vi "ExeCmd_CallCollect.vi"(4 "HighPrio":bool, 6 "CmdVIRef":refnum<vi>, 7 "ActorClassObjectIn":refnum<class>, 8 "ErrorIn":errorcluster, 9 "NameOfVi2Call(optional)":string, 10 "CmdData":variant, 11 "YActorIn":refnum<class "YActor.lvclass">) -> (0 "ErrorOut":errorcluster, 2 "ReplyData":variant, 5 "ActorClassObjectOut":refnum<class>)   [LabVIEW 2021, in "YActor.lvclass"]
uses:
  YActor.lvclass
  YActor.lvclass/YActor.ctl
  private/CmdCtrl.ctl
  AsyncErrorHandling.ctl
  private/CallMode.ctl
  InlineReferencePool.ctl
panel:
  # "Do not use this VI in a loop where different Cmd VI references are routed.\nThis will cause the execution of the first called command VI only"
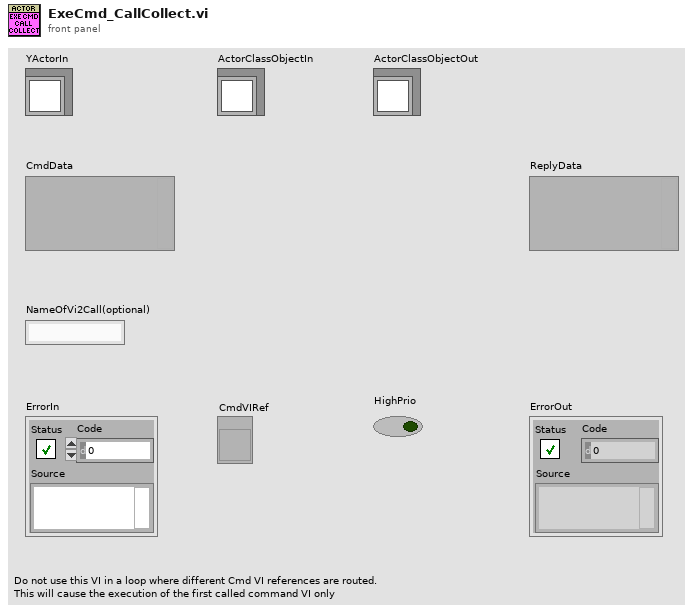
[diagram p1: front panel]
types:
  T1 = typedef "YActor.lvclass/CallMode.ctl" = enum16{"Standard", "Call&Collect"}
  T2 = typedef "YActor.lvclass/InlineReferencePool.ctl" = enum16{"Add", "ClearAll?"}
  T3 = typedef "YActor.lvclass/CmdCtrl.ctl" = cluster{"CmdData":variant, "CommandVI":string, "ReplyQ":i64, "Error":errorcluster, "Msg#":u32, "AsyncErrorHandling":T4, "CallMode":T1, "Source":string}
  T4 = typedef "YActor.lvclass/AsyncErrorHandling.ctl" = enum16{"Return after executing sync command", "Return before executing sync command", "Don't return error"}
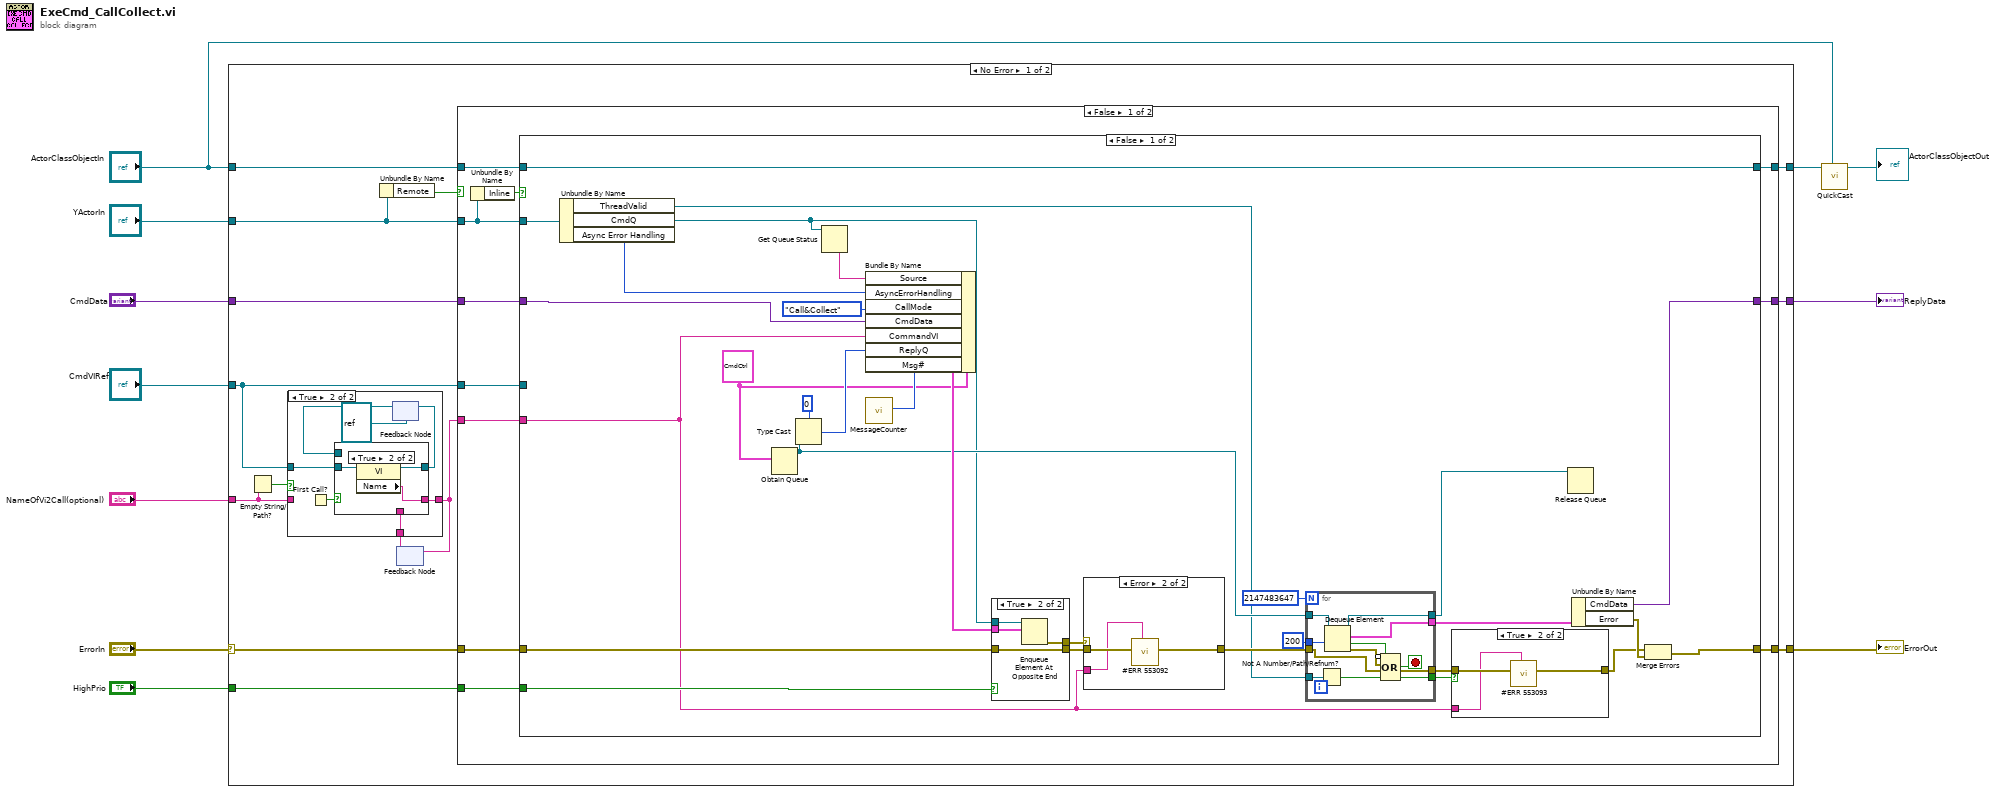
[diagram p0: block diagram]
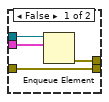
[diagram p6: hidden frame]
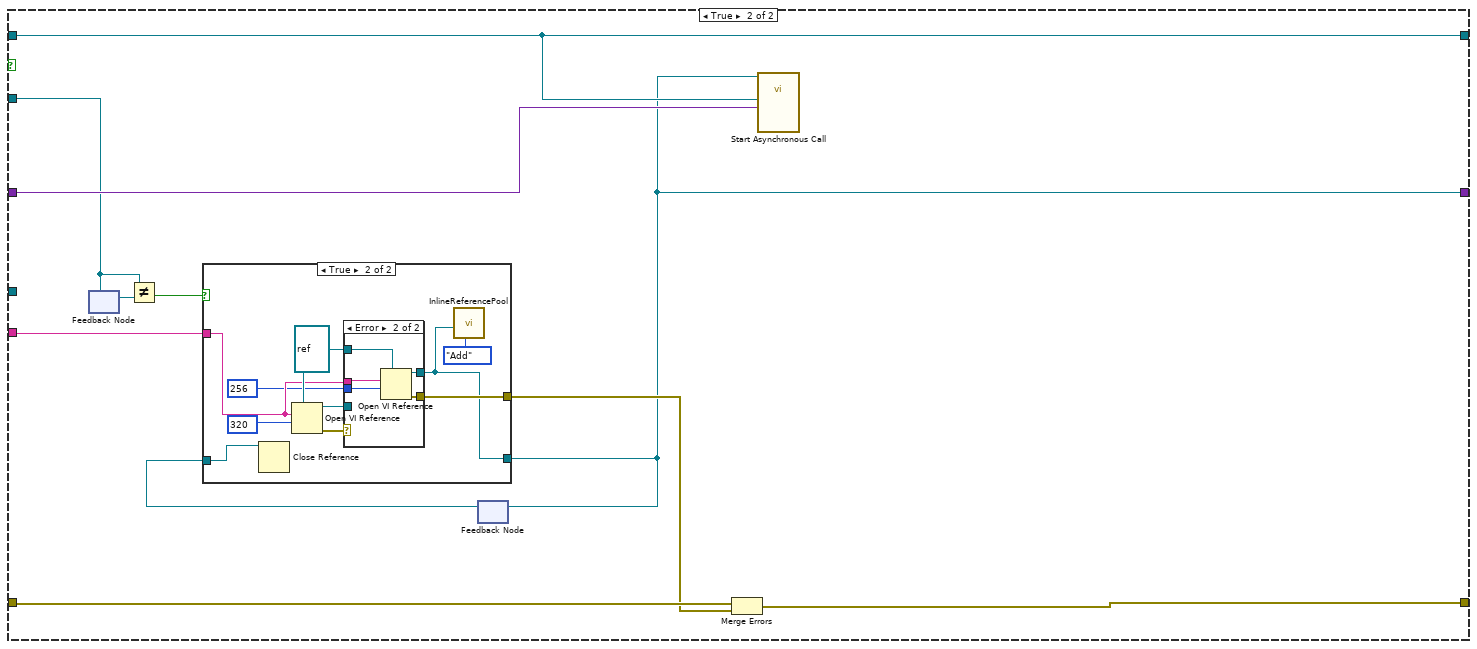
[diagram p7: hidden frame]
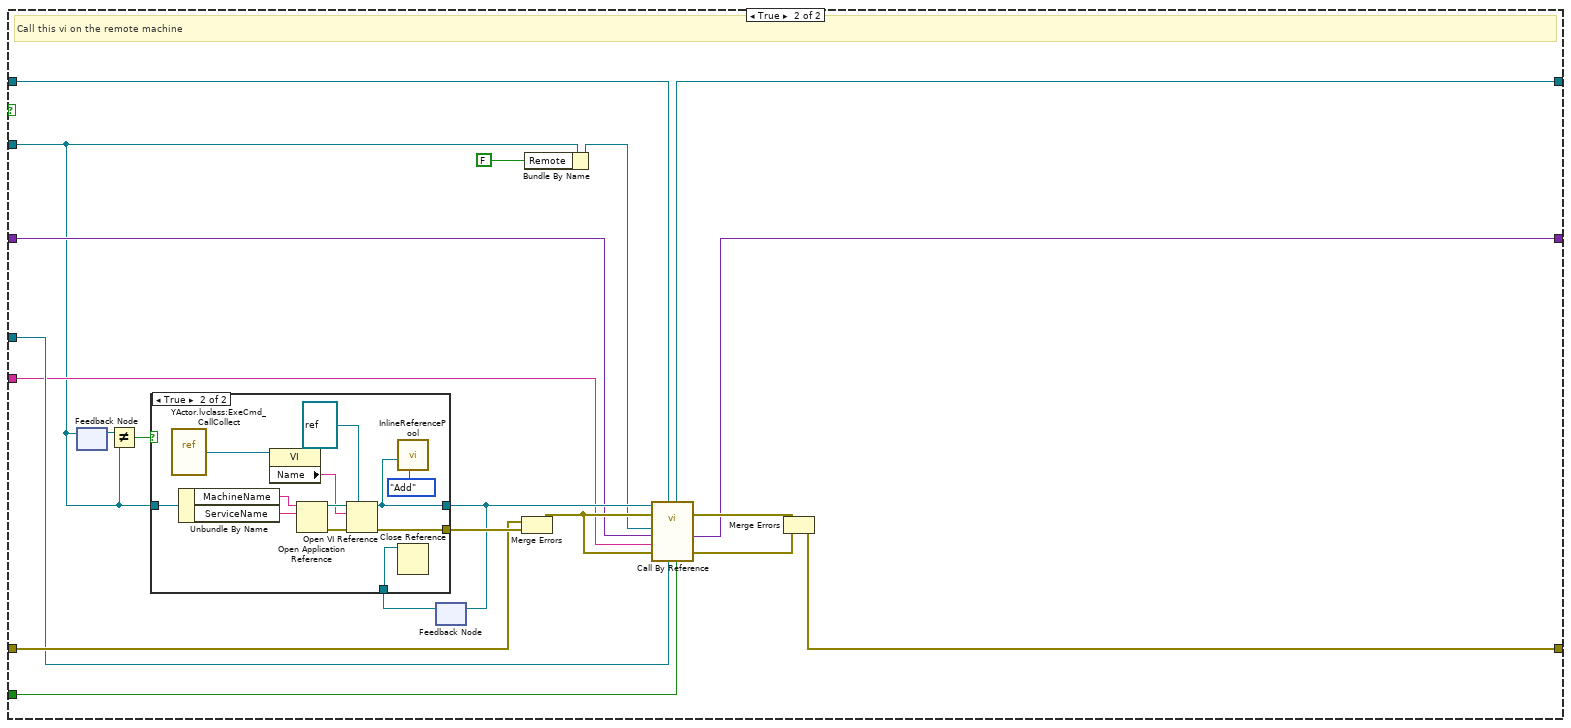
[diagram p10: hidden frame]
diagram:
  n1 = case shown="No Error" "ErrorIn" {
    selector: "ErrorIn" -> [w24 w170]
    tunnel: [w25 w170] -> w10
    tunnel: "YActorIn" -> [w18 _]
    tunnel: "CmdData" -> [w21 w169]
    tunnel: "CmdVIRef" -> [w15 _]
    tunnel: [w23 w169] -> w6
    tunnel: "HighPrio" -> [w22 _]
    tunnel: "ActorClassObjectIn" -> [w19 w168]
    tunnel: [w20 w168] -> w3
    tunnel: "NameOfVi2Call(optional)" -> [w13 _]
    frame No Error {
      n2 = Empty String/Path?(string/path=w13) -> (empty?=w12:bool)
      n3 = Unbundle By Name(w18) -> ("Remote"=w17:bool)
      n4 = feedback #1() -> (w16:string)  [unwired: 1 in]
      n5 = case shown="True" w12 {
        tunnel: w16 -> [_ w31]
        tunnel: [w26 w30] -> w14
        tunnel: w15 -> [_ w29]
        tunnel: w13 -> [w26 _]
        frame False {
        }
        frame True {
          n6 = First Call?() -> (First Call?: T/F=w27:bool)
          n7 = feedback #2(refnum<vi> refnum ("Cmd VI ref")) -> (w28:refnum<vi>)
          n8 = case shown="True" w27 {
            tunnel: w29 -> [_ w38]
            tunnel: [w35 w37] -> w30
            tunnel: w31 -> [w35 _]
            tunnel: [w34 w36] -> w32
            tunnel: w28 -> [w34 _]
            frame False {
            }
            frame True {
              n9 = property class="VI"(reference=w38) -> (reference out=w36:refnum<vi>, "Name"=w37:string)  [unwired: 1 in, 1 out]
            }
          }
          n10 = feedback-in #2(w32) -> ()
        }
      }
      n11 = feedback-in #1(w14) -> ()
      n12 = case shown="False" w17 {
        tunnel: [w47 w140] -> w23
        tunnel: [w49 w149] -> w25
        tunnel: w24 -> [w48 w153]
        tunnel: w22 -> [w46 w142]
        tunnel: w21 -> [w45 w139]
        tunnel: w15 -> [w44 w143]
        tunnel: w18 -> [w43 w136]
        tunnel: w19 -> [w41 w146]
        tunnel: [w40 w141] -> w20
        tunnel: w14 -> [w39 w138]
        frame False {
          n13 = Unbundle By Name(w43) -> ("Inline"=w42:bool)
          n14 = case shown="False" w42 {
            tunnel: [w69 w109] -> w47
            tunnel: [w79 w115] -> w49
            tunnel: w48 -> [w78 w116]
            tunnel: w46 -> [w67 _]
            tunnel: w45 -> [w64 w110]
            tunnel: w44 -> [_ _]
            tunnel: w43 -> [w55 w107]
            tunnel: w41 -> [w54 w111]
            tunnel: [w54 w111] -> w40
            tunnel: w39 -> [w53 w113]
            frame False {
              w50 = T3 {"CmdData"=variant(refnum<class> refnum), "CommandVI"="", "ReplyQ"=0, "Error"={"Status"=FALSE, "Code"=0, "Source"=""}, "Msg#"=0, "AsyncErrorHandling"=enum."Return after executing sync command", "CallMode"=enum."Standard", "Source"=""} ("CmdCtrl")
              n15 = Unbundle By Name(w55) -> ("ThreadValid"=w65:refnum<queue>, "CmdQ"=w52:refnum<queue>, "Async Error Handling"=w56:T4)
              n16 = Obtain Queue(element data type=w50) -> (queue out=w68:refnum<queue>)  [unwired: 4 in, 2 out]
              n17 = Type Cast(type=i64 0, x=w68) -> (*(type *) &x=w71:i64)
              n18 = Get Queue Status(queue=w52) -> (queue name=w51:string)  [unwired: 2 in, 7 out]
              n19 = call "MessageCounter.vi"() -> ("Msg#"=w66:u32)  [unwired: 11 in]
              n20 = Bundle By Name(cluster=w50, "Source"=w51, "AsyncErrorHandling"=w56, "CallMode"=CallMode."Call&Collect", "CmdData"=w64, "CommandVI"=w53, "ReplyQ"=w71, "Msg#"=w66) -> (w70:T3)
              n21 = case shown="True" w67 {
                tunnel: w52 -> [w99 w103]
                tunnel: w70 -> [w98 w102]
                tunnel: [w101 w105] -> w77
                tunnel: w78 -> [w100 w104]
                tunnel: [w100 w104] -> w76
                frame False {
                  n22 = Enqueue Element(queue=w99, element=w98) -> (error out=w101:errorcluster)  [unwired: 2 in, 2 out]
                }
                frame True {
                  n23 = Enqueue Element At Opposite End(queue=w103, element=w102) -> (error out=w105:errorcluster)  [unwired: 2 in, 2 out]
                }
              }
              n24 = case shown="Error" w77 {
                tunnel: w76 -> [w94 w96]
                tunnel: [w94 w97] -> w75
                tunnel: w53 -> [_ w95]
                frame No Error {
                }
                frame Error {
                  n25 = call "#ERR 553092"("Data"=w95, "error in (no error)"=w96) -> ("error out"=w97:errorcluster)  [unwired: 9 in]
                }
              }
              n26 = for {
                N: 2147483647 -> [_]
                tunnel: [w91] -> w62
                tunnel: w65 -> [w85]
                tunnel: 200 -> [w87]
                tunnel: w75 -> [w92]
                tunnel: w68 -> [w90]
                tunnel: [w89] -> w61
                tunnel: [w92] -> w73
                tunnel: [w84] -> w58
                stop <- w88 stop-if-true
                n27 = Not A Number/Path/Refnum?(number/path/refnum=w85) -> (NaN/Path/Refnum?=w84:bool)
                n28 = Dequeue Element(queue=w90, timeout in ms (-1)=w87) -> (queue out=w89:refnum<queue>, element=w91:T3, timed out?=w86:bool, error out=w93:errorcluster)  [unwired: 1 in]
                n29 = Compound Arithmetic op=OR(invert w86, w93, w92, w84) -> (w88:bool)
              }
              n30 = case shown="True" w58 {
                tunnel: w73 -> [w80 w83]
                tunnel: w53 -> [_ w81]
                tunnel: [w80 w82] -> w72
                frame False {
                }
                frame True {
                  n31 = call "#ERR 553093"("Data"=w81, "error in (no error)"=w83) -> ("error out"=w82:errorcluster)  [unwired: 9 in]
                }
              }
              n32 = Release Queue(queue=w61) -> ()  [unwired: 2 in, 3 out]
              n33 = Unbundle By Name(w62) -> ("CmdData"=w69:variant, "Error"=w74:errorcluster)
              n34 = Merge Errors(w72, w74) -> (w79:errorcluster)
            }
            frame True {
              n35 = feedback #3() -> (w108:refnum<class "YActor.lvclass">)  [unwired: 1 in]
              n36 = feedback-in #3(w107) -> ()
              n37 = Not Equal?(x=w107, y=w108) -> (x != y?=w106:bool)
              n38 = feedback #4() -> (w112:refnum<vi>)  [unwired: 1 in]
              n39 = case shown="True" w106 {
                tunnel: [w117 w121] -> w109
                tunnel: w112 -> [w117 w118]
                tunnel: w113 -> [_ w123]
                tunnel: [_ w126] -> w114
                frame False {
                }
                frame True {
                  w125 = refnum<vi> refnum ("type specifier VI Refnum (for type only)")
                  n40 = Close Reference(reference=w118) -> ()  [unwired: 1 in, 1 out]
                  n41 = Open VI Reference(type specifier VI Refnum (for type only)=w125, vi path=w123, options=320) -> (vi reference=w124:refnum<vi>, error out=w127:errorcluster)  [unwired: 3 in]
                  n42 = case shown="Error" w127 {
                    selector: w127 -> [w129 _]
                    tunnel: w123 -> [_ w133]
                    tunnel: w125 -> [_ w132]
                    tunnel: [w128 w131] -> w121
                    tunnel: [w129 w134] -> w126
                    tunnel: w124 -> [w128 _]
                    tunnel: 256 ("options") -> [_ w130]
                    frame No Error {
                    }
                    frame Error {
                      n43 = Open VI Reference(type specifier VI Refnum (for type only)=w132, vi path=w133, options=w130) -> (vi reference=w131:refnum<vi>, error out=w134:errorcluster)  [unwired: 3 in]
                    }
                  }
                  n44 = call "InlineReferencePool.vi"("Functions"=InlineReferencePool."Add" ("functions"), "InlineViRef"=w121) -> ()  [unwired: 8 in, 2 out]
                }
              }
              n45 = feedback-in #4(w109) -> ()
              n46 = Merge Errors(w116, w114) -> (w115:errorcluster)
              n47 = call-by-ref "Start Asynchronous Call"(reference=w109, "Cmd Data"=w110, "Local in"=w111) -> ()  [unwired: 7 in, 6 out]
            }
          }
        }
        frame True {
          # "Call this vi on the remote machine"
          n48 = feedback-in #5(w136) -> ()
          n49 = feedback #5() -> (w137:refnum<class "YActor.lvclass">)  [unwired: 1 in]
          n50 = Not Equal?(x=w137, y=w136) -> (x != y?=w135:bool)
          n51 = feedback #6() -> (w147:refnum<vi>)  [unwired: 1 in]
          n52 = case shown="True" w135 {
            tunnel: w136 -> [_ w164]
            tunnel: [w155 w158] -> w148
            tunnel: w147 -> [w155 w156]
            tunnel: [_ w166] -> w154
            frame False {
            }
            frame True {
              n53 = vi-ref "YActor.lvclass:ExeCmd_CallCollect.vi"() -> (w165:refnum<vi>)
              n54 = Unbundle By Name(w164) -> ("MachineName"=w163:string, "ServiceName"=w162:string)
              n55 = property class="VI"(reference=w165) -> ("Name"=w160:string)  [unwired: 1 in, 2 out]
              n56 = Open Application Reference(10:w162, 11:w163) -> (0:w167:errorcluster, 3:w161:refnum<vi>)  [unwired: 2 in]
              n57 = Open VI Reference(type specifier VI Refnum (for type only)=refnum<vi> refnum, application reference (local)=w161, vi path=w160, error in (no error)=w167) -> (vi reference=w158:refnum<vi>, error out=w166:errorcluster)  [unwired: 2 in]
              n58 = call "InlineReferencePool.vi"("Functions"=InlineReferencePool."Add" ("functions"), "InlineViRef"=w158) -> ()  [unwired: 8 in, 2 out]
              n59 = Close Reference(reference=w156) -> ()  [unwired: 1 in, 1 out]
            }
          }
          n60 = feedback-in #6(w148) -> ()
          n61 = Merge Errors(w153, w154) -> (w152:errorcluster)
          n62 = Bundle By Name(cluster=w136, "Remote"=FALSE ("Remote.Remote?")) -> (w145:refnum<class "YActor.lvclass">)
          n63 = call-by-ref "?"(reference=w148, error in=w152, "High Prio"=w142, "Cmd VI ref"=w143, "ActorClass object in"=w146, 8:"error in (no error)"=w152, "NameOfVi2Call (optional)"=w138, "Cmd Data"=w139, "reference in"=w145) -> (error out=w151:errorcluster, 0:"error out"=w150:errorcluster, "Reply Data"=w140:variant, "ActorClass object out"=w141:refnum<class>)  [unwired: 2 in, 1 out]
          n64 = Merge Errors(w151, w150) -> (w149:errorcluster)
        }
      }
    }
    frame Error {
    }
  }
  "ErrorOut" <- w10
  "ReplyData" <- w6
  n65 = call "QuickCast.vi"("YActorIn"=w3, "ObjectTargetType"="ActorClassObjectIn") -> ("ObjectOut"=→"ActorClassObjectOut":refnum<class>)  [unwired: 9 in]
